vi "LaunchCC.vi"() -> ()   [LabVIEW 2014]
panel:
  out "Recently Opened File Names":string[](array[string])
  out "VI Name 2":string
  out "error out 3":errorcluster
  out "Application:Exported VIs In Memory":string[](array[string])
  out "Application:Version Year":string
  out "Application:Active:VI":string
  out "error out 4":errorcluster
  out "error out 2":errorcluster
  out "VI Path":path
  out "VI Name":string
  out "error out":errorcluster
  out "OpenDyna":errorcluster
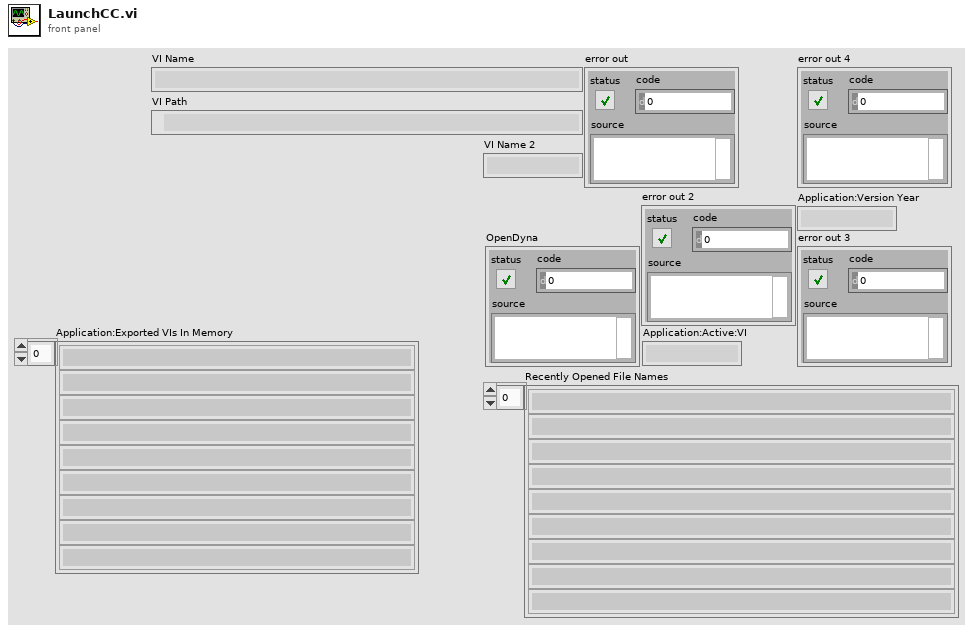
[diagram p1: front panel]
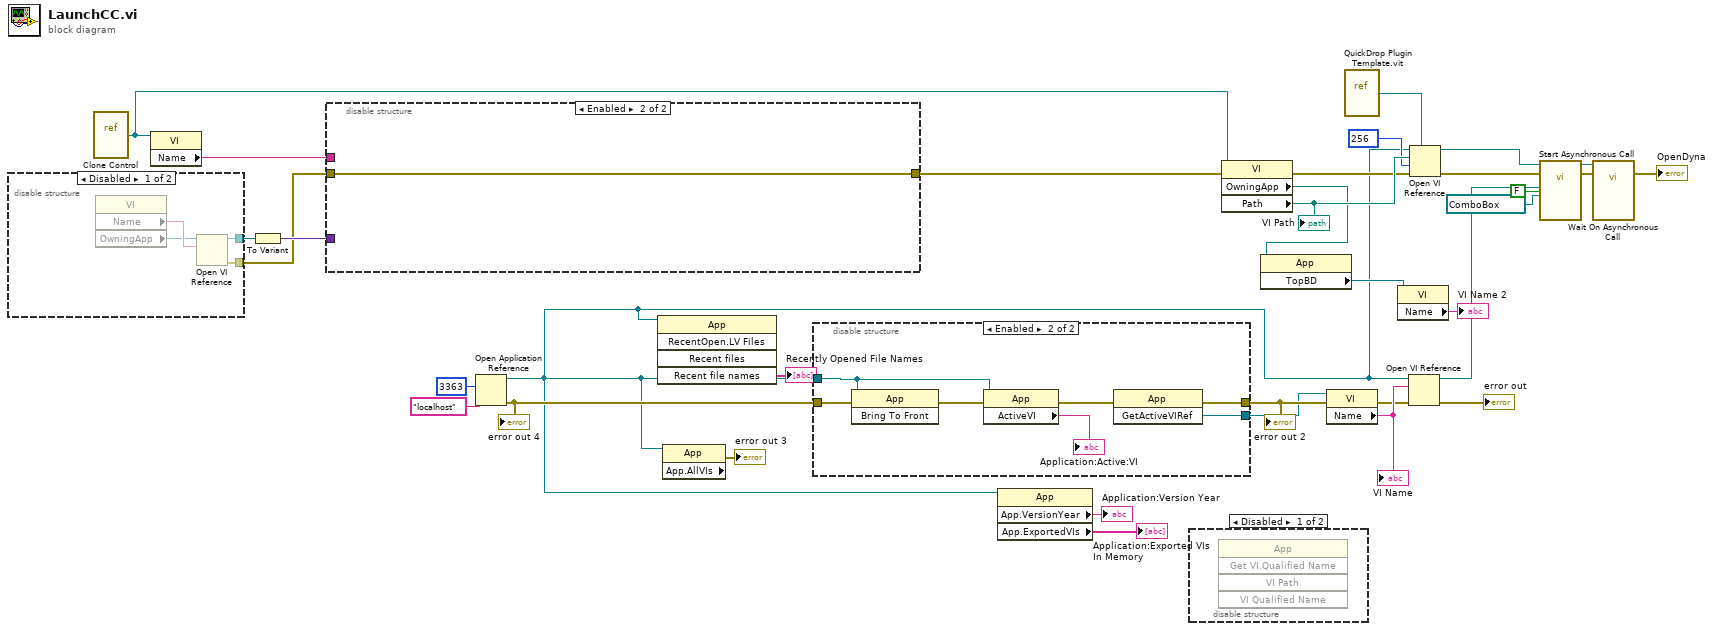
[diagram p0: block diagram]
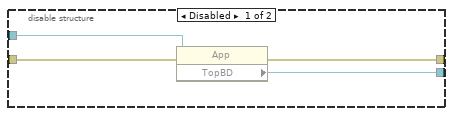
[diagram p3: hidden frame]
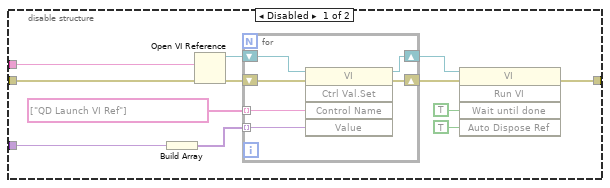
[diagram p5: hidden frame]
diagram:
  n1 = disable-structure shown="Disabled" {
    disable-tunnel: [w37 _] -> w32
    disable-tunnel: [w36 _] -> w10
    frame Disabled {
      n2 = property class="VI"() -> (reference=w35:refnum<vi>, "Name"=w39:string, "OwningApp"=w38:refnum<vi>)  [unwired: 1 in, 2 out]
      n3 = Open VI Reference(application reference (local)=w38, vi path=w39) -> (vi reference=w36:refnum<vi>, error out=w37:errorcluster)  [unwired: 4 in]
    }
    frame Enabled {
    }
  }
  n4 = vi-ref <resource>:"Clone Control.vi"() -> (w19:refnum<vi>)
  n5 = property class="VI"(reference=w19) -> ("Name"=w33:string)  [unwired: 1 in, 2 out]
  n6 = To Variant(anything=w10) -> (Variant=w34:variant)
  n7 = disable-structure shown="Enabled" {
    disable-tunnel: w34 -> [w47 _]
    disable-tunnel: w33 -> [w44 _]
    disable-tunnel: w32 -> [w43 w58]
    disable-tunnel: [w42 w58] -> w23
    frame Disabled {
      n8 = Build Array(w47) -> (w46:variant[])
      n9 = Open VI Reference(vi path=w44, error in (no error)=w43) -> (vi reference=w48:refnum<vi>, error out=w49:errorcluster)  [unwired: 1 in, 3 out]
      n10 = for {
        shift-right: [w55] -> w50
        shift-left: w49 -> [w56]
        shift-right: [w54] -> w51
        shift-left: w48 -> [w57]
        tunnel: string[] ["QD Launch VI Ref"] ("ParamNames") -> [w53] mode=indexing
        tunnel: w46 -> [w52] mode=indexing
        n11 = invoke class="VI" method="Ctrl Val.Set"(reference=w57, error in=w56, "Control Name"=w53, "Value"=w52) -> (reference out=w54:refnum<vi>, error out=w55:errorcluster)  [unwired: 1 in, 3 out]
      }
      n12 = invoke class="VI" method="Run VI"(reference=w51, error in=w50, "Wait until done"=TRUE ("Wait Until Done"), "Auto Dispose Ref"=TRUE ("Auto Dispose Reference")) -> (error out=w42:errorcluster)  [unwired: 1 in, 4 out]
    }
    frame Enabled {
    }
  }
  n13 = Open Application Reference(10:u16 3363 ("port number or service name (3363)"), 11:"localhost" ("machine name (\"\":  open local reference)")) -> (0:w15:errorcluster, 3:w3:refnum<vi>)  [unwired: 2 in]
  "error out 4" <- w15
  n14 = invoke class="App" method="RecentOpen.LV Files"(reference=w3) -> ("Recent file names"=→"Recently Opened File Names":string[])  [unwired: 4 in, 4 out]
  n15 = property class="App" props=["App.AllVIs"](reference=w3) -> (error out=→"error out 3":errorcluster)  [unwired: 1 in, 2 out]
  n16 = disable-structure shown="Enabled" {
    disable-tunnel: w15 -> [w62 w65]
    disable-tunnel: w3 -> [w61 w67]
    disable-tunnel: [w60 w63] -> w14
    disable-tunnel: [w59 w68] -> w12
    frame Disabled {
      n17 = property class="App"(reference=w61, error in=w62) -> (error out=w60:errorcluster, "TopBD"=w59:refnum<vi>)  [unwired: 1 out]
    }
    frame Enabled {
      n18 = invoke class="App" method="Bring To Front"(reference=w67, error in=w65) -> (error out=w66:errorcluster)  [unwired: 1 in, 2 out]
      n19 = property class="App"(reference=w67, error in=w66) -> (error out=w64:errorcluster, "ActiveVI"=→"Application:Active:VI":string)  [unwired: 1 out]
      n20 = invoke class="App" method="GetActiveVIRef"(error in=w64) -> (error out=w63:errorcluster, "GetActiveVIRef"=w68:refnum<vi>)  [unwired: 2 in, 1 out]
    }
  }
  "error out 2" <- w14
  n21 = property class="App"(reference=w3) -> ("App.VersionYear"=→"Application:Version Year":string, "App.ExportedVIs"=→"Application:Exported VIs In Memory":string[])  [unwired: 1 in, 2 out]
  n22 = disable-structure shown="Disabled" {
    frame Disabled {
      n23 = invoke class="App" method="Get VI.Qualified Name"() -> ()  [unwired: 5 in, 5 out]
    }
    frame Enabled {
    }
  }
  n24 = property class="VI"(reference=w19, error in=w23) -> (error out=w26:errorcluster, "OwningApp"=w6:refnum<vi>, "Path"=w31:path)  [unwired: 1 out]
  "VI Path" <- w31
  n25 = property class="App"(reference=w6) -> ("TopBD"=w5:refnum<vi>)  [unwired: 1 in, 2 out]
  n26 = property class="VI"(reference=w12, error in=w14) -> (error out=w13:errorcluster, "Name"=w17:string)  [unwired: 1 out]
  "VI Name" <- w17
  n27 = vi-ref <resource>:"QuickDrop Plugin Template.vit"() -> (w25:refnum<vi>)
  n28 = property class="VI"(reference=w5) -> ("Name"=→"VI Name 2":string)  [unwired: 1 in, 2 out]
  n29 = Open VI Reference(application reference (local)=w3, vi path=w17, error in (no error)=w13) -> (vi reference=w9:refnum<vi>, error out=→"error out":errorcluster)  [unwired: 3 in]
  n30 = Open VI Reference(type specifier VI Refnum (for type only)=w25, application reference (local)=w3, vi path=w31, options=256, error in (no error)=w26) -> (vi reference=w30:refnum<vi>, error out=w20:errorcluster)  [unwired: 1 in]
  n31 = call-by-ref "Start Asynchronous Call"(reference=w30, error in=w20, "Shift Pressed?"=FALSE, "QD Combo Box Ref"=refnum<vi> refnum, "QD Launch VI Ref"=w9) -> (reference out=w24:refnum<vi>, error out=w22:errorcluster)  [unwired: 7 in, 2 out]
  n32 = call-by-ref "Wait On Asynchronous Call"(reference=w24, error in=w22) -> (error out=→"OpenDyna":errorcluster)  [unwired: 10 in, 3 out]
